vi "FPGA Main.vi"() -> ()   [LabVIEW 2022 SP3]
uses:
  <vilib>/rvi/Emulation/niFpgaGetClockAttributes.vi
  <vilib>/rvi/Emulation/niFpgaSctlEmulationGetInTimedLoop.vi
  <vilib>/rvi/Emulation/niFpgaEmulationReportErrorSimple.vi
  <vilib>/rvi/eio/common/nirviEmuTemplateMethod_errors.vi
  <vilib>/rvi/Emulation/niFpgaCriticalErrorInLSC.vi
  <vilib>/eio/EIONode/EIONode.xnode
panel:
  out "波形图表 3":sgl(graph)
  out "波形图表 2":sgl(graph)
  out "波形图表":sgl(graph)
  in  "模块7/User LED":bool
  in  "模块7/Phase B Pos":bool
  in  "模块7/Phase A Pos":bool
  in  "模块7/Phase B Neg":bool
  in  "模块7/Phase A Neg":bool
  out "模块7/Vsup Voltage":u16
  out "模块7/Phase B Current":i16
  out "模块7/Phase A Current":i16
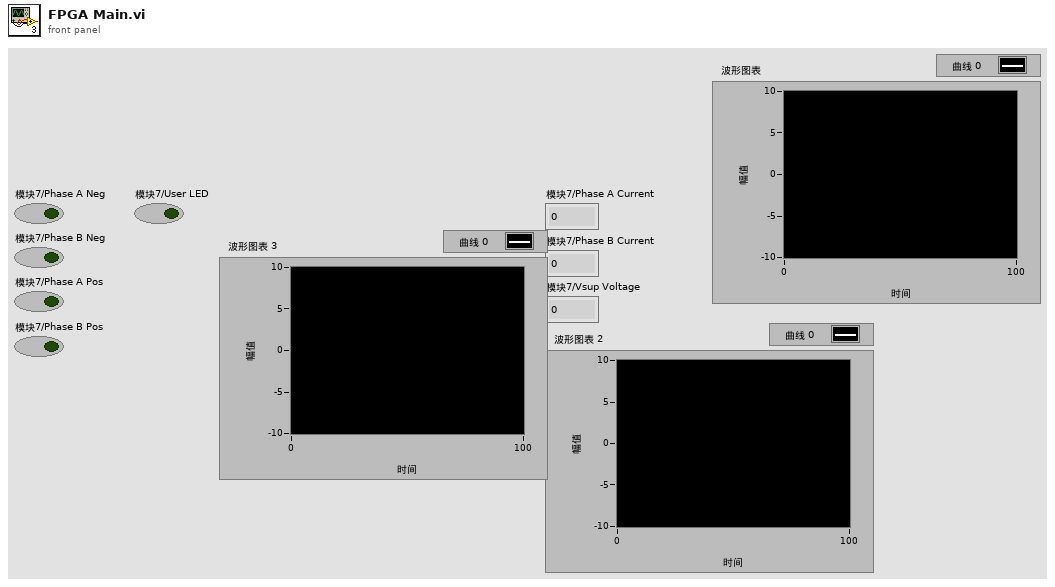
[diagram p1: front panel]
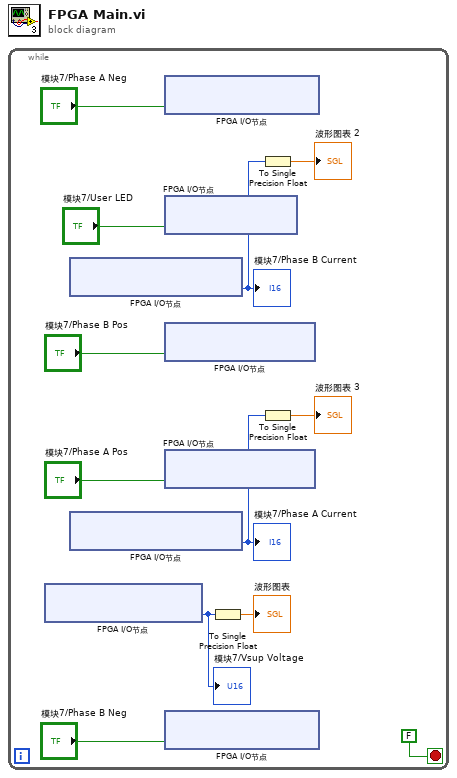
[diagram p0: block diagram]
diagram:
  n1 = while {
    stop <- FALSE stop-if-true
    n2 = xnode "FPGA I/O节点"() -> ("模块7/Vsup Voltage"=w6:u16)  [unwired: 1 in, 1 out]
    "模块7/Vsup Voltage" <- w6
    n3 = xnode "FPGA I/O节点"() -> ("模块7/Phase B Current"=w2:i16)  [unwired: 1 in, 1 out]
    "模块7/Phase B Current" <- w2
    n4 = xnode "FPGA I/O节点"() -> ("模块7/Phase A Current"=w1:i16)  [unwired: 1 in, 1 out]
    "模块7/Phase A Current" <- w1
    n5 = xnode "FPGA I/O节点"("模块7/Phase A Neg"="模块7/Phase A Neg") -> ()  [unwired: 1 in, 1 out]
    n6 = xnode "FPGA I/O节点"("模块7/User LED"="模块7/User LED") -> ()  [unwired: 1 in, 1 out]
    n7 = xnode "FPGA I/O节点"("模块7/Phase B Pos"="模块7/Phase B Pos") -> ()  [unwired: 1 in, 1 out]
    n8 = xnode "FPGA I/O节点"("模块7/Phase A Pos"="模块7/Phase A Pos") -> ()  [unwired: 1 in, 1 out]
    n9 = xnode "FPGA I/O节点"("模块7/Phase B Neg"="模块7/Phase B Neg") -> ()  [unwired: 1 in, 1 out]
    n10 = To Single Precision Float(number=w6) -> (single precision float=→"波形图表":sgl)
    n11 = To Single Precision Float(number=w2) -> (single precision float=→"波形图表 2":sgl)
    n12 = To Single Precision Float(number=w1) -> (single precision float=→"波形图表 3":sgl)
  }
